vi "polcal_new.vi"(7 "LCVR variable":T1, 8 "ErrorOut":errorcluster, 9 "file path (dialog if empty)":path, 10 "BuffNr":i16, 11 "ph":u64) -> (0 "ErrorOut 2":errorcluster, 3 "hout":u64)   [LabVIEW 2014]
uses:
  <vilib>/Platform/TimedLoop/XDataNode/timing_clust.ctl
  <vilib>/Platform/TimedLoop/XDataNode/nitl_modes.ctl
  <vilib>/Platform/TimedLoop/XDataNode/wakeup.ctl
  gfitsio/cfitsio-bitpix.ctl
  <vilib>/platform/TimedLoop/XDataNode/XDataNode.xnode
  <userlib>/Newport ESP301/Newport ESP301.lvlib
  <vilib>/Platform/TimedLoop/XDataNode/XDNodeRunTimeDep.lvlib
  gfitsio/gfitsio.lvlib
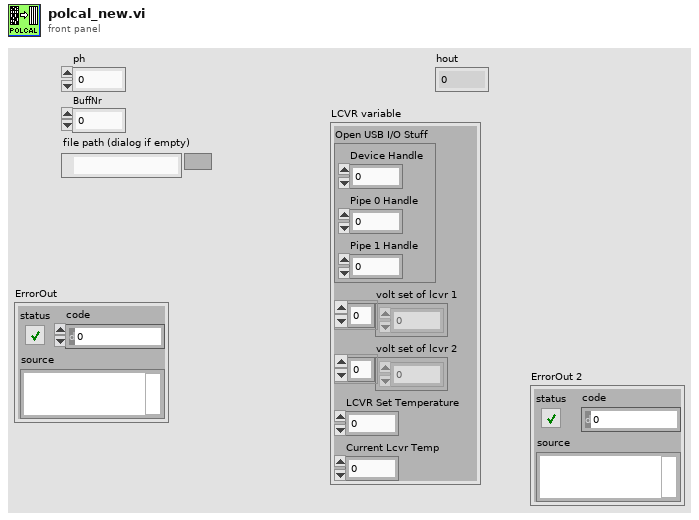
[diagram p1: front panel]
types:
  T1 = cluster{"Open USB I/O Stuff":cluster{"Device Handle":u32, "Pipe 0 Handle":u32, "Pipe 1 Handle":u32}, "volt set of lcvr 1":dbl[], "volt set of lcvr 2":dbl[], "LCVR Set Temperature":dbl, "Current Lcvr Temp":dbl}
  T2 = enum16{"Find +0 Position Count", "Find Home and Index Signals", "Find Home Signal", "Find Positive Limit Signal", "Find Negative Limit Signal", "Find Positve Limit and Index Signals", "Find Negative Limit and Index Signals"}
  T3 = typedef "XDNodeRunTimeDep.lvlib/timing_clust.ctl" = cluster{"Expected End [f-1]":u64, "Actual End [f-1]":u64, "Finished Late? [f-1]":bool, "Expected End [i-1]":u64, "Actual End [i-1]":u64, "Finished Late? [i-1]":bool, "Expected Start [i]":u64, "Actual Start [i]":u64, "Expected Start [f]":u64, "Actual Start [f]":u64, "Source Name":string, "Structure Name":string, "Period":i64, "Deadline":i64, "Offset":i64, "Start":i64, "Priority":i32, "Timeout":i32, "Mode":T4, "Wakeup Reason":T5, "Error":errorcluster, "Source Type":string, "Secondary Source Type":string, "Global End Time":u64, "Global Start Time":u64, "Frame Duration":u64, "Iteration Duration":u64, "Assigned CPU":i32, "I/O Scan Engine Mode":u32}
  T4 = typedef "XDNodeRunTimeDep.lvlib/nitl_modes.ctl" = enum32{"No Change", "Process missed periods, maintain original phase", "Discard missed periods, maintain original phase", "Process missed periods, ignore original phase", "Discard missed periods, ignore original phase"}
  T5 = typedef "XDNodeRunTimeDep.lvlib/wakeup.ctl" = enum32{"Normal", "Aborted", "Asynchronous wakeup", "Timing source error", "Timed loop error", "Timeout"}
  T6 = cluster{"Device Handle":u32, "Pipe 0 Handle":u32, "Pipe 1 Handle":u32}
  T7 = enum16{"open", "open or create", "create or replace", "create", "open (read only)"}
  T8 = typedef "gfitsio.lvlib/cfitsio-bitpix.ctl" = i32
  T9 = typedef "gfitsio.lvlib/gfitsio-refnum.ctl" = refnum<k1>
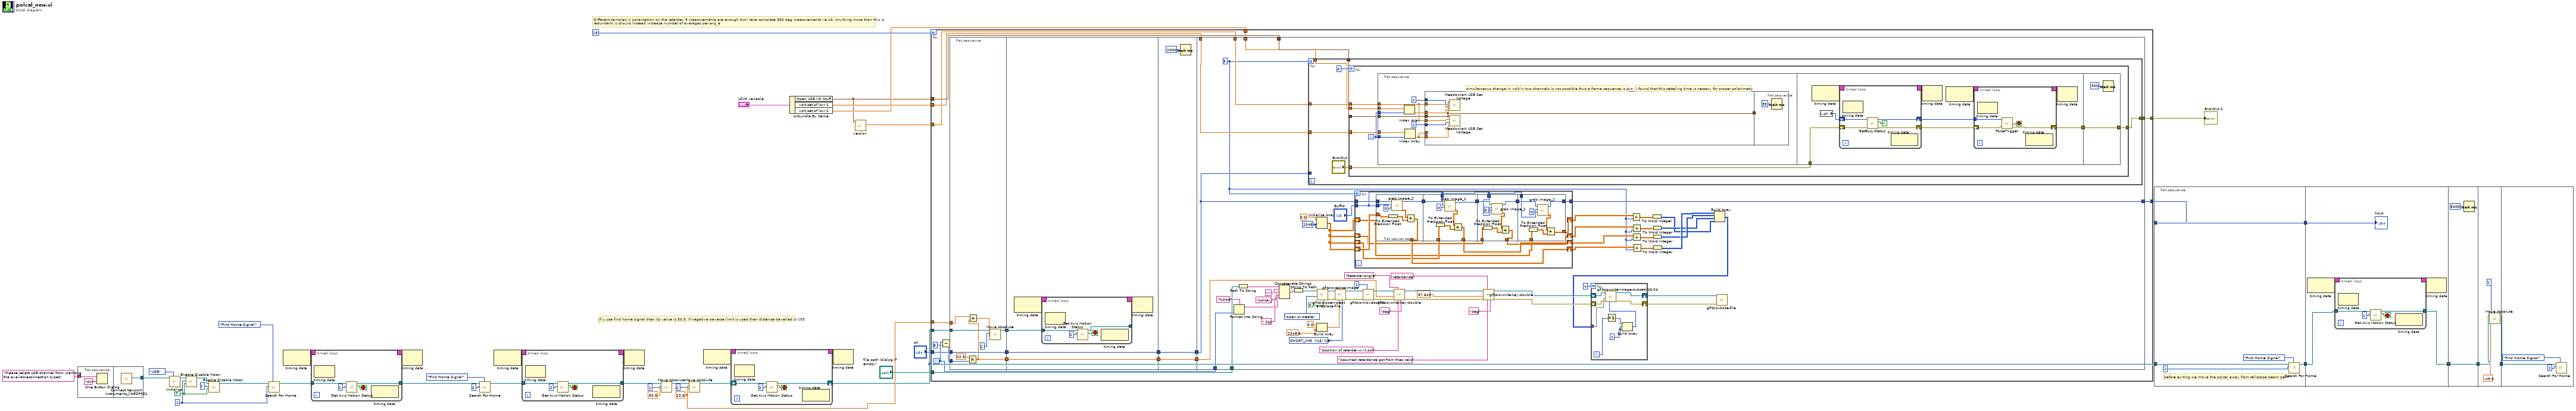
[diagram p0: block diagram]
diagram:
  w4 = 23.6 ("Position (0 units)")
  w40 = TRUE ("Action (F - OFF)")
  w37 = 1 ("Axis (1)")
  # "."
  # "If u use find home signal then its value is 50.5. If negative traverse limit is used then distance travelled is 103"
  # "."
  # "Different samples in polarisation on the retarder. 8 measurements are enough but I take complete 360 deg measurements i;e 16. Anything more than this is \nredundant. U should instead increase number of averages per angle"
  n1 = flat-sequence {
    tunnel: "Please select USB channel from \namong the availableconnection types" ("message") -> [w46]
    tunnel: [w47] -> w19
    frame #0 {
      n2 = One Button Dialog(message=w46, button name ("OK")="OK") -> ()  [unwired: 1 out]
    }
    frame #1 {
      n3 = call <userlib>:"Connect Newport Instruments_libESP301.vi"() -> ("VISA resource name (duplicate)"=w47:refnum<visa-resource-name>)  [unwired: 7 in, 4 out]
    }
  }
  n4 = call <userlib>:"Initialize.vi"("VISA resource name"=w19, "Serial Link (RS232)"=enum16{"RS232", "USB"}."USB") -> ("VISA resource name out"=w43:refnum<visa-resource-name>)  [unwired: 7 in, 1 out]
  n5 = call <userlib>:"Enable Disable Motor.vi"("Action (F - OFF)"=w40, "Axis (1)"=w37, "VISA resource name"=w43) -> ("VISA resource name out"=w42:refnum<visa-resource-name>)  [unwired: 3 in, 1 out]
  n6 = call <userlib>:"Enable Disable Motor.vi"("Action (F - OFF)"=w40, "Axis (1)"=2, "VISA resource name"=w42) -> ("VISA resource name out"=w39:refnum<visa-resource-name>)  [unwired: 3 in, 1 out]
  n7 = call <userlib>:"Search For Home.vi"("Home mode"=T2."Find Home Signal", "Axis (1)"=w37, "VISA resource name"=w39) -> ("VISA resource name out"=w34:refnum<visa-resource-name>)  [unwired: 4 in, 1 out]
  n8 = node-c288() -> (w36:T3)  [unwired: 1 in]
  n9 = timed-loop {
    timing: w36 -> [_]
    timing-out: [_] -> w35
    tunnel: w34 -> [w50]
    tunnel: [w48] -> w33
    stop <- w51 stop-if-true
    n10 = node-c288() -> ()  [unwired: 1 in, 1 out]
    n11 = call <userlib>:"Get Axis Motion Status.vi"("Axis (1)"=1, "VISA resource name"=w50) -> ("Motion Done"=w51:bool, "VISA resource name out"=w48:refnum<visa-resource-name>)  [unwired: 3 in, 1 out]
    n12 = node-c288() -> ()  [unwired: 1 in, 1 out]
  }
  n13 = node-c288(w35) -> ()  [unwired: 1 out]
  n14 = call <userlib>:"Search For Home.vi"("Home mode"=T2."Find Home Signal", "Axis (1)"=2, "VISA resource name"=w33) -> ("VISA resource name out"=w28:refnum<visa-resource-name>)  [unwired: 4 in, 1 out]
  n15 = node-c288() -> (w30:T3)  [unwired: 1 in]
  n16 = timed-loop {
    timing: w30 -> [_]
    timing-out: [_] -> w29
    tunnel: w28 -> [w56]
    tunnel: [w54] -> w17
    stop <- w57 stop-if-true
    n17 = node-c288() -> ()  [unwired: 1 in, 1 out]
    n18 = call <userlib>:"Get Axis Motion Status.vi"("Axis (1)"=2, "VISA resource name"=w56) -> ("Motion Done"=w57:bool, "VISA resource name out"=w54:refnum<visa-resource-name>)  [unwired: 3 in, 1 out]
    n19 = node-c288() -> ()  [unwired: 1 in, 1 out]
  }
  n20 = node-c288(w29) -> ()  [unwired: 1 out]
  n21 = call <userlib>:"Move Absolute.vi"("Position (0 units)"=50.5, "Axis (1)"=1, "VISA resource name"=w17) -> ("VISA resource name out"=w14:refnum<visa-resource-name>)  [unwired: 3 in, 1 out]
  n22 = call <userlib>:"Move Absolute.vi"("Position (0 units)"=w4, "Axis (1)"=2, "VISA resource name"=w14) -> ("VISA resource name out"=w24:refnum<visa-resource-name>)  [unwired: 3 in, 1 out]
  n23 = node-c288() -> (w26:T3)  [unwired: 1 in]
  n24 = timed-loop {
    timing: w26 -> [_]
    timing-out: [_] -> w25
    shift-right: [w60] -> w3
    shift-left: w24 -> [w62]
    stop <- w63 stop-if-true
    n25 = node-c288() -> ()  [unwired: 1 in, 1 out]
    n26 = call <userlib>:"Get Axis Motion Status.vi"("Axis (1)"=2, "VISA resource name"=w62) -> ("Motion Done"=w63:bool, "VISA resource name out"=w60:refnum<visa-resource-name>)  [unwired: 3 in, 1 out]
    n27 = node-c288() -> ()  [unwired: 1 in, 1 out]
  }
  n28 = Unbundle By Name("LCVR variable") -> ("Open USB I/O Stuff"=w8:T6, "volt set of lcvr 1"=w10:dbl[], "volt set of lcvr 2"=w9:dbl[])
  n29 = node-c288(w25) -> ()  [unwired: 1 out]
  n30 = call "version.vi"("USB Open Device Cluster"=w8) -> ("Version"=w7:dbl)  [unwired: 10 in]
  n31 = for {
    N: 15 -> [_]
    tunnel: "ph" -> [w85]
    tunnel: "file path (dialog if empty)" -> [w76]
    tunnel: w3 -> [w83]
    tunnel: [w75] -> w18
    tunnel: w8 -> [w74]
    tunnel: w10 -> [w73]
    tunnel: w9 -> [w72]
    tunnel: w7 -> [w71]
    tunnel: [w70] -> w6
    tunnel: w4 -> [w69]
    i -> [w68]
    n32 = Subtract(x=w68, y=8) -> (x-y=w66:i32)
    n33 = flat-sequence {
      tunnel: w85 -> [w94]
      tunnel: [w94] -> w84
      tunnel: w83 -> [w93]
      tunnel: w66 -> [w91]
      tunnel: [w89] -> w80
      tunnel: [w87] -> w79
      tunnel: w69 -> [w88]
      tunnel: w84 -> [w99]
      tunnel: [w99] -> w82
      tunnel: w80 -> [w96]
      tunnel: w79 -> [w95]
      tunnel: [w95] -> w77
      tunnel: w82 -> [w110]
      tunnel: [w110] -> w81
      tunnel: [w108] -> w78
      tunnel: w77 -> [w108]
      tunnel: w81 -> [w169]
      tunnel: w78 -> [w153]
      tunnel: w76 -> [w142]
      tunnel: w68 -> [w138]
      tunnel: [w132] -> w75
      tunnel: w74 -> [w131]
      tunnel: w73 -> [w130]
      tunnel: w72 -> [w129]
      tunnel: w71 -> [w128]
      tunnel: [w127] -> w70
      frame #0 {
        n34 = Multiply(x=22.5, y=w91) -> (x*y=w87:dbl)
        n35 = Add(x=w88, y=w87) -> (x+y=w86:dbl)
        n36 = call <userlib>:"Move Absolute.vi"("Position (0 units)"=w86, "Axis (1)"=2, "VISA resource name"=w93) -> ("VISA resource name out"=w89:refnum<visa-resource-name>)  [unwired: 3 in, 1 out]
      }
      frame #1 {
        n37 = node-c288() -> (w98:T3)  [unwired: 1 in]
        n38 = timed-loop {
          timing: w98 -> [_]
          timing-out: [_] -> w97
          tunnel: w96 -> [w102]
          tunnel: [w100] -> _
          stop <- w103 stop-if-true
          n39 = node-c288() -> ()  [unwired: 1 in, 1 out]
          n40 = call <userlib>:"Get Axis Motion Status.vi"("Axis (1)"=2, "VISA resource name"=w102) -> ("Motion Done"=w103:bool, "VISA resource name out"=w100:refnum<visa-resource-name>)  [unwired: 3 in, 1 out]
          n41 = node-c288() -> ()  [unwired: 1 in, 1 out]
        }
        n42 = node-c288(w97) -> ()  [unwired: 1 out]
      }
      frame #2 {
        n43 = Wait (ms)(milliseconds to wait=u32 2000) -> ()  [unwired: 1 out]
      }
      frame #3 {
        w165 = T8 16 items=["<invalid type>"=0, "BYTE_IMG  (U8)"=8, "SHORT_IMG  (I16)"=16, "USHORT_IMG  (U16)"=20, "LONG_IMG  (I32)"=32, "ULONG_IMG  (U32)"=40, "FLOAT_IMG  (SGL)"=-32, "DOUBLE_IMG  (DBL)"=-64] ("image data type")
        w167 = 2048.0 ("element")
        w172 = 2048 ("dimension size")
        w119 = 5
        n44 = Format Into String(format string="%04d", w138) -> (resulting string=w136:string)  [unwired: 2 in, 1 out]
        n45 = Path To String(path=w142) -> (string=w141:string)
        n46 = Concatenate Strings(w141, "\\" ("string"), "polcal_" ("string"), w136, ".fits" ("string")) -> (w135:string)
        n47 = String To Path(string=w135) -> (path=w134:path)
        n48 = for {
          N: w119 -> [_]
          tunnel: w169 -> [_]
          tunnel: w131 -> [w234]
          tunnel: w130 -> [w233]
          tunnel: w129 -> [w232]
          tunnel: w128 -> [w231]
          tunnel: [w229] -> w127
          n49 = for {
            N: 4 -> [_]
            tunnel: "ErrorOut" -> [w242]
            tunnel: [w241] -> w229
            tunnel: w234 -> [w240]
            tunnel: w233 -> [w239]
            tunnel: w232 -> [w238]
            tunnel: w231 -> [w237]
            i -> [w243]
            n50 = flat-sequence {
              tunnel: w237 -> [w247]
              tunnel: w238 -> [w251]
              tunnel: w239 -> [w252]
              tunnel: w240 -> [w250]
              tunnel: w243 -> [w254]
              tunnel: w243 -> [w253]
              tunnel: w242 -> [w269]
              tunnel: [w268] -> w236
              tunnel: [w290] -> w241
              tunnel: w236 -> [w290]
              frame #0 {
                # "simultaneous change in volt in two channels is not possible thus a frame sequence is put"
                # "I found that this setteling time is nessary for proper polarimetry"
                n51 = Index Array(array=w251, index=w254) -> (element=w248:dbl)
                n52 = Index Array(array=w252, index=w253) -> (element=w244:dbl)
                n53 = flat-sequence {
                  tunnel: [w261] -> w245
                  tunnel: w244 -> [w258]
                  tunnel: w247 -> [w260]
                  tunnel: 1 ("LC Channel") -> [w259]
                  tunnel: w244 -> [_]
                  tunnel: w250 -> [w261]
                  tunnel: w247 -> [w257]
                  tunnel: 2 ("LC Channel") -> [w256]
                  tunnel: w248 -> [w255]
                  tunnel: w245 -> [_]
                  frame #0 {
                    n54 = call "Meadowlark USB Set Voltage.VI"("LC Voltage"=w255, "LC Channel"=w256, "FW Version"=w257, "USB Open Device Cluster"=w261) -> ()  [unwired: 1 out]
                    n55 = call "Meadowlark USB Set Voltage.VI"("LC Voltage"=w258, "LC Channel"=w259, "FW Version"=w260, "USB Open Device Cluster"=w261) -> ()  [unwired: 1 out]
                  }
                  frame #1 {
                    n56 = Wait (ms)(milliseconds to wait=u32 35) -> ()  [unwired: 1 out]
                  }
                }
              }
              frame #1 {
                n57 = node-c288() -> (w267:T3)  [unwired: 1 in]
                n58 = local read "ph"() -> (w263:u64)
                n59 = timed-loop {
                  shift-right: [w281] -> w271
                  shift-left: w263 -> [w284]
                  shift-right: [w282] -> w270
                  shift-left: w269 -> [w283]
                  timing: w267 -> [_]
                  timing-out: [_] -> w266
                  stop <- w280 continue-if-true
                  n60 = node-c288() -> ()  [unwired: 1 in, 1 out]
                  n61 = call <userlib>:"GetBusyStatus.vi"("error in (no error)"=w283, "ph"=w284) -> ("error out"=w282:errorcluster, "BusyState"=w280:bool, "hout"=w281:u64)  [unwired: 2 in, 1 out]
                  n62 = node-c288() -> ()  [unwired: 1 in, 1 out]
                }
                n63 = node-c288(w266) -> ()  [unwired: 1 out]
                n64 = node-c288() -> (w265:T3)  [unwired: 1 in]
                n65 = timed-loop {
                  tunnel: w271 -> [w275]
                  shift-right: [w272] -> w268
                  shift-left: w270 -> [w273]
                  timing: w265 -> [_]
                  timing-out: [_] -> w264
                  stop <- w274 stop-if-true
                  n66 = node-c288() -> ()  [unwired: 1 in, 1 out]
                  n67 = call <userlib>:"ForceTrigger.vi"("ph"=w275, "error in (no error)"=w273) -> ("Triggered"=w274:bool, "error out"=w272:errorcluster)  [unwired: 1 in, 2 out]
                  n68 = node-c288() -> ()  [unwired: 1 in, 1 out]
                }
                n69 = node-c288(w264) -> ()  [unwired: 1 out]
              }
              frame #2 {
                n70 = Wait (ms)(milliseconds to wait=u32 300) -> ()  [unwired: 1 out]
              }
            }
          }
        }
        n71 = Initialize Array(0.0 ("element"), w172, w172) -> (w124:dbl[][])
        n72 = Build Array(4.0 ("element"), w167, w167) -> (w166:dbl[])
        n73 = call "gfitsio-open-create-replace-file.vi"("advisory dialog? (display:T)"=FALSE, "function (open)"=T7."open or create", "file path (dialog if empty)"=w134) -> ("error out"=w162:errorcluster, "gfits refnum"=w168:T9)  [unwired: 6 in, 1 out]
        n74 = call "gfitsio-resize-image.vi"("image data type"=w165, "naxes"=w166, "error in (no error)"=w162, "gfits refnum"=w168) -> ("error out"=w157:errorcluster, "dup gfits refnum"=w158:T9)  [unwired: 6 in]
        n75 = for {
          N: w119 -> [_]
          tunnel: "BuffNr" -> [w186]
          tunnel: w169 -> [w196]
          shift-right: [w192] -> w170
          shift-left: w124 -> [w195]
          tunnel: [w194] -> w132
          shift-right: [w191] -> w125
          shift-left: w124 -> [w190]
          shift-right: [w188] -> w121
          shift-left: w124 -> [w183]
          shift-right: [w185] -> w120
          shift-left: w124 -> [w184]
          n76 = flat-sequence {
            tunnel: w186 -> [w203]
            tunnel: w196 -> [w202]
            tunnel: w195 -> [w201]
            tunnel: [w198] -> w193
            tunnel: [w197] -> w192
            tunnel: w193 -> [w212]
            tunnel: w186 -> [w209]
            tunnel: [w206] -> w191
            tunnel: w190 -> [w205]
            tunnel: [w211] -> w189
            tunnel: w189 -> [w217]
            tunnel: w186 -> [w215]
            tunnel: [w214] -> w188
            tunnel: [w216] -> w187
            tunnel: w183 -> [w213]
            tunnel: [w224] -> w194
            tunnel: w187 -> [w225]
            tunnel: w186 -> [w223]
            tunnel: [w222] -> w185
            tunnel: w184 -> [w221]
            frame #0 {
              n77 = To Extended Precision Float(1:w201) -> (0:w200:ext[][])
              n78 = call "grab image_2.vi"("Image number"=u32 0, "BuffNr"=w203, "ph"=w202) -> ("output image"=w199:dbl[][], "hout"=w198:u64)  [unwired: 5 in, 2 out]
              n79 = Add(x=w199, y=w200) -> (x+y=w197:ext[][])
            }
            frame #1 {
              n80 = To Extended Precision Float(1:w205) -> (0:w208:ext[][])
              n81 = call "grab image_2.vi"("Image number"=u32 0, "BuffNr"=w209, "ph"=w212) -> ("output image"=w207:dbl[][], "hout"=w211:u64)  [unwired: 5 in, 2 out]
              n82 = Add(x=w207, y=w208) -> (x+y=w206:ext[][])
            }
            frame #2 {
              n83 = To Extended Precision Float(1:w213) -> (0:w219:ext[][])
              n84 = call "grab image_2.vi"("Image number"=u32 0, "BuffNr"=w215, "ph"=w217) -> ("output image"=w218:dbl[][], "hout"=w216:u64)  [unwired: 5 in, 2 out]
              n85 = Add(x=w218, y=w219) -> (x+y=w214:ext[][])
            }
            frame #3 {
              n86 = To Extended Precision Float(1:w221) -> (0:w227:ext[][])
              n87 = call "grab image_2.vi"("Image number"=u32 0, "BuffNr"=w223, "ph"=w225) -> ("output image"=w226:dbl[][], "hout"=w224:u64)  [unwired: 5 in, 2 out]
              n88 = Add(x=w226, y=w227) -> (x+y=w222:ext[][])
            }
          }
        }
        n89 = call "gfitsio-movabs-hdu.vi"("hdunum"=1, "error in (no error)"=w157, "gfits refnum"=w158) -> ("error out"=w145:errorcluster, "dup gfits refnum"=w155:T9)  [unwired: 6 in, 1 out]
        n90 = call "gfitsio-write-key-double.vi"("units"="deg", "comment"="position of retarder w.r.t pol", "keyname"="Retarder angle", "error in (no error)"=w145, "value"=w153, "gfits refnum"=w155) -> ("error out"=w144:errorcluster, "dup gfits refnum"=w151:T9)  [unwired: 4 in]
        n91 = call "gfitsio-write-key-double.vi"("units"="deg", "comment"="Assumed retardance got from theo calc", "keyname"="retardance", "error in (no error)"=w144, "value"=87.643, "gfits refnum"=w151) -> ("error out"=w143:errorcluster, "dup gfits refnum"=w146:T9)  [unwired: 4 in]
        n92 = Divide(x=w120, y=w119) -> (x/y=w122:ext[][])
        n93 = Divide(x=w121, y=w119) -> (x/y=w123:ext[][])
        n94 = Divide(x=w125, y=w119) -> (x/y=w126:ext[][])
        n95 = Divide(x=w170, y=w119) -> (x/y=w161:ext[][])
        n96 = To Word Integer(number=w122) -> (16bit integer=w115:i16[][])
        n97 = To Word Integer(number=w123) -> (16bit integer=w116:i16[][])
        n98 = To Word Integer(number=w126) -> (16bit integer=w117:i16[][])
        n99 = To Word Integer(number=w161) -> (16bit integer=w118:i16[][])
        n100 = Build Array(w118, w117, w116, w115) -> (w112:i16[][][])
        n101 = for {
          N: 4 -> [_]
          shift-right: [w182] -> w160
          shift-left: w146 -> [w180]
          shift-right: [w181] -> w159
          shift-left: w143 -> [w179]
          tunnel: w112 -> [w174] mode=indexing
          i -> [w178]
          w176 = 1 ("element")
          n102 = Increment(x=w178) -> (x+1=w177:i32)
          n103 = Build Array(w177, w176, w176) -> (w175:i32[])
          n104 = call "gfitsio-write-image-subset-i16-2d.vi"("fpixel"=w175, "error in (no error)"=w179, "data"=w174, "gfits refnum"=w180) -> ("error out"=w181:errorcluster, "dup gfits refnum"=w182:T9)  [unwired: 6 in]
        }
        n105 = call "gfitsio-close-file.vi"("error in (no error)"=w159, "gfits refnum"=w160) -> ()  [unwired: 8 in, 2 out]
      }
    }
  }
  "ErrorOut 2" <- w6
  n106 = flat-sequence {
    tunnel: w18 -> [w295]
    tunnel: w3 -> [w293]
    tunnel: [w295] -> w13
    tunnel: [w291] -> w12
    tunnel: w13 -> [w300]
    tunnel: w12 -> [w297]
    tunnel: [w296] -> w2
    tunnel: w2 -> [w310]
    tunnel: [w310] -> w1
    tunnel: w1 -> [w314]
    tunnel: [w311] -> w5
    tunnel: w5 -> [w317]
    frame #0 {
      # "before exiting we move the polcal away from teliscope beam path"
      n107 = call <userlib>:"Search For Home.vi"("Home mode"=T2."Find Home Signal", "Axis (1)"=1, "VISA resource name"=w293) -> ("VISA resource name out"=w291:refnum<visa-resource-name>)  [unwired: 4 in, 1 out]
    }
    frame #1 {
      n108 = node-c288() -> (w299:T3)  [unwired: 1 in]
      n109 = timed-loop {
        timing: w299 -> [_]
        timing-out: [_] -> w298
        tunnel: w297 -> [w303]
        tunnel: [w301] -> w296
        stop <- w304 stop-if-true
        n110 = node-c288() -> ()  [unwired: 1 in, 1 out]
        n111 = call <userlib>:"Get Axis Motion Status.vi"("Axis (1)"=1, "VISA resource name"=w303) -> ("Motion Done"=w304:bool, "VISA resource name out"=w301:refnum<visa-resource-name>)  [unwired: 3 in, 1 out]
        n112 = node-c288() -> ()  [unwired: 1 in, 1 out]
      }
      n113 = node-c288(w298) -> ()  [unwired: 1 out]
      "hout" <- w300
    }
    frame #2 {
      n114 = Wait (ms)(milliseconds to wait=u32 3000) -> ()  [unwired: 1 out]
    }
    frame #3 {
      n115 = call <userlib>:"Move Absolute.vi"("Position (0 units)"=-49.0, "Axis (1)"=1, "VISA resource name"=w314) -> ("VISA resource name out"=w311:refnum<visa-resource-name>)  [unwired: 3 in, 1 out]
    }
    frame #4 {
      n116 = call <userlib>:"Search For Home.vi"("Home mode"=T2."Find Home Signal", "Axis (1)"=2, "VISA resource name"=w317) -> ()  [unwired: 4 in, 2 out]
    }
  }
